vi "9. CoffeeMaker Documentation.vi"(6 "Simulation":cluster{"Water":dbl, "Coffee":dbl, "Milk":dbl} caption="Wasser" {"Milk" step=1.0 scale=0.0..100.0; "Water" step=1.0 scale=0.0..100.0; "Coffee" step=1.0 scale=0.0..100.0}, 7 "Power Switch":bool, 11 "Coffee Selection":T2 caption="Selection" {"Type" min=0 max=2 step=1 scale=0.0..2.0}) -> (0 "error out":errorcluster, 3 "Display":T1 {"Coffee" scale=0.0..80.0; "Brewing Chamber" scale=0.0..80.0})   [LabVIEW 2018]
doc: "Coffee Machine Version 1.0: final solution. Extensive documentation and VI appearance added"
uses:
  Controls/States.ctl
  <vilib>/Utility/miscctls.llb/LVMinMaxIncTypeDef.ctl
  <vilib>/Utility/file.llb/Read Delimited Spreadsheet (DBL).vi
  <vilib>/Utility/file.llb/Read Delimited Spreadsheet (string).vi
  <vilib>/Utility/file.llb/Write Delimited Spreadsheet (DBL).vi
panel:
  out "s? t:f":enum16{"next state", "current state"}(ring)
  # "CLD Coffee Machine v1.0"
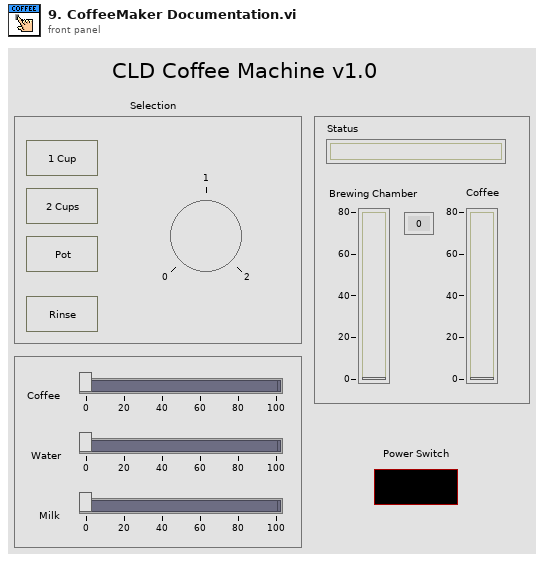
[diagram p1: front panel]
types:
  T1 = cluster{"Brewing Chamber":i8, "Coffee":i8, "Status":string, "Remaining Time:":i32}
  T2 = cluster{"1 Cup":bool, "2 Cups":bool, "Pot":bool, "Rinse":bool, "Type":i8}
  T3 = cluster{"Status":refnum<vi>, "Brewing Chamber":refnum<vi>, "Coffee":refnum<vi>, "Power Switch":refnum<vi>}
  T4 = enum8{"Enabled", "Disabled", "Disabled and Grayed Out"}
  T5 = typedef "LVMinMaxIncTypeDef.ctl" = cluster{"Minimum":dbl, "Maximum":dbl, "Increment":dbl}
  T6 = typedef "States.ctl" = enum16{"Initialize", "Set Language", "Wait for Power On", "Heat up", "Check and Wait for Water", "Rinsing", "Check Resources", "User Input", "Grinding", "Boiling", "Pouring", "Rinse before Stop", "Write Data", "Stop"}
  T7 = cluster{"Coffee":refnum<vi>, "Water":refnum<vi>, "Milk":refnum<vi>}
  T8 = cluster{"Coffee Selection":refnum<vi>, "1 Cup":refnum<vi>, "2 Cups":refnum<vi>, "Pot":refnum<vi>, "Rinse":refnum<vi>, "Type":refnum<vi>}
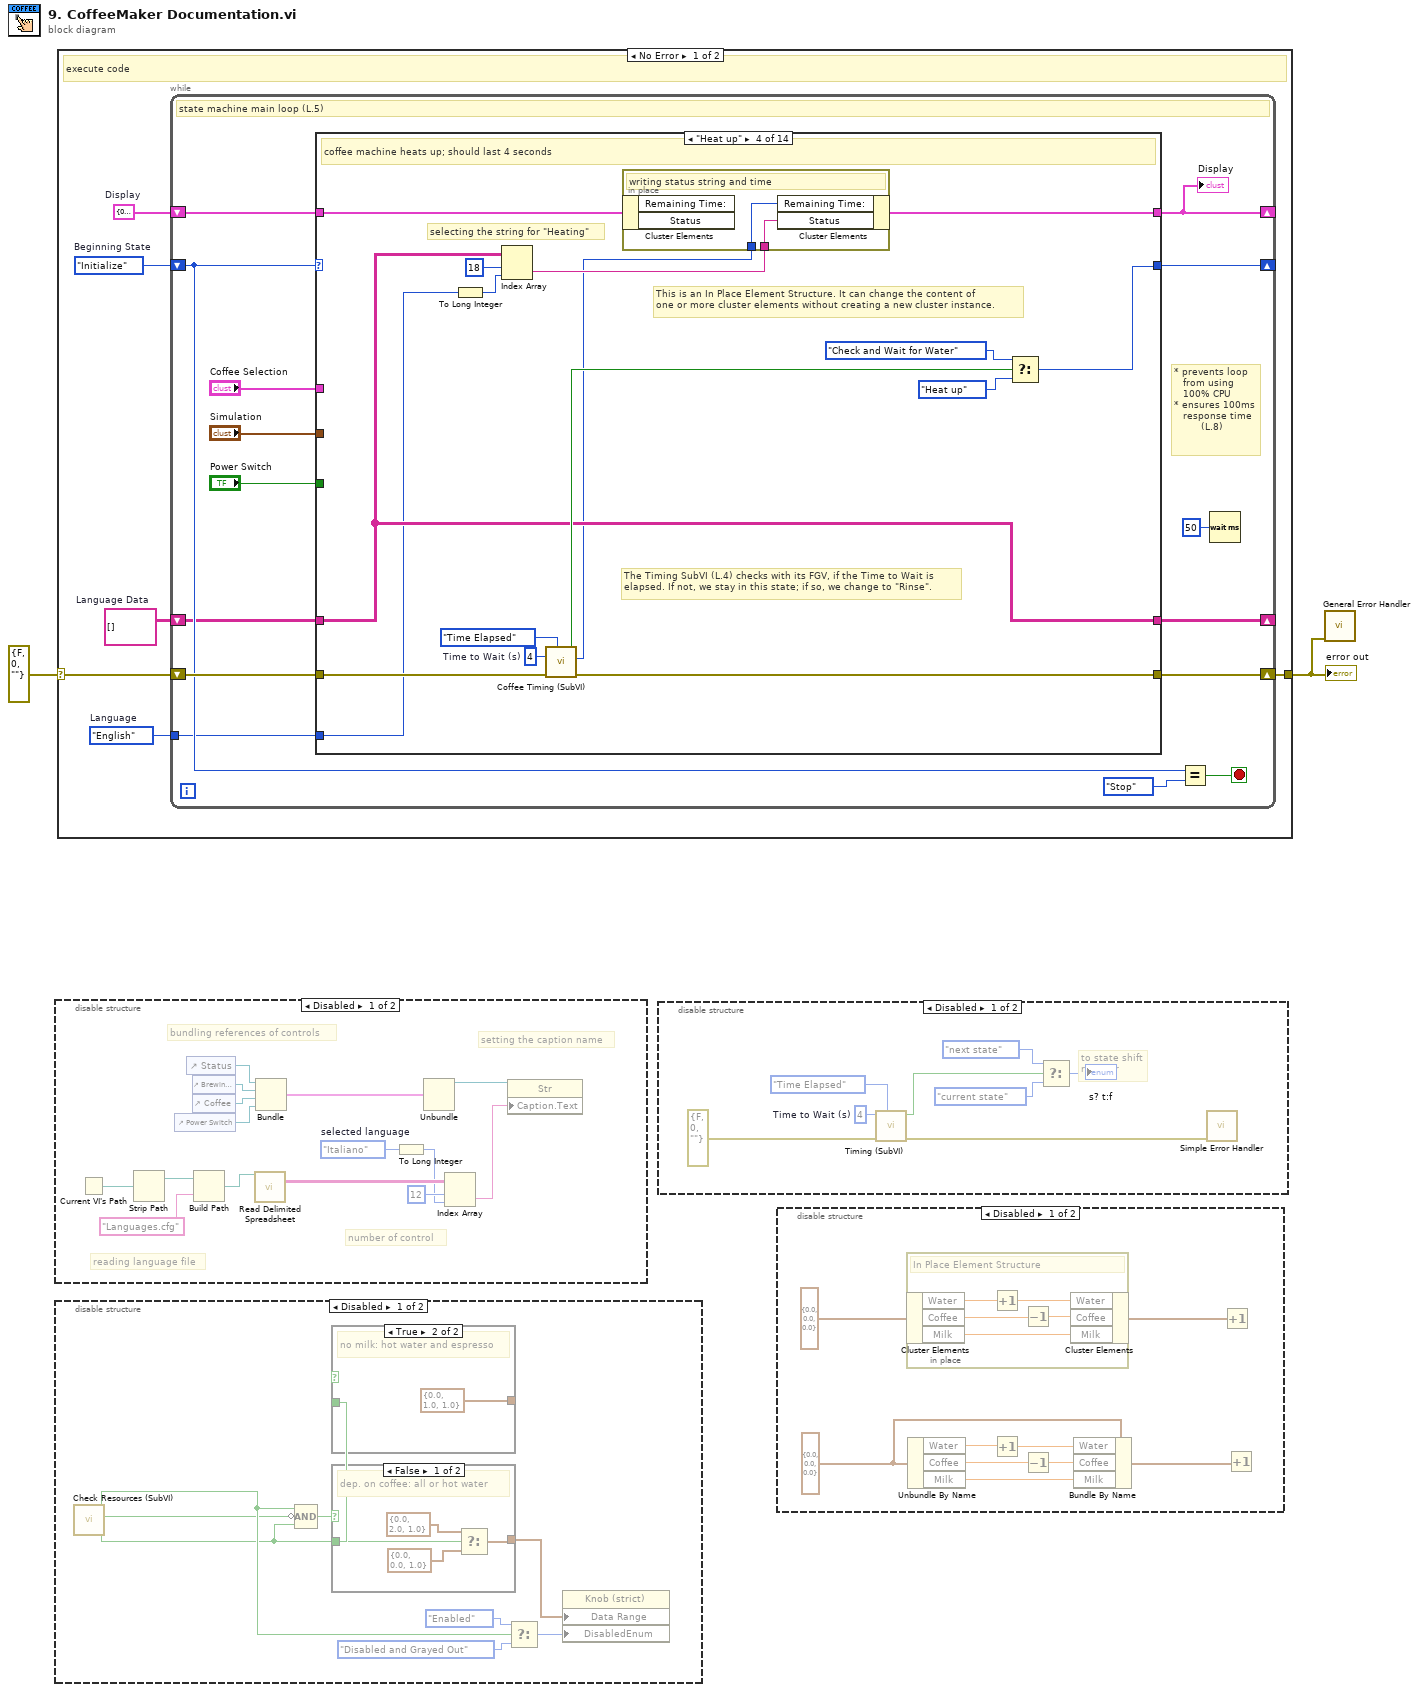
[diagram p0: block diagram]
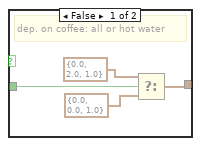
[diagram p3: hidden frame]
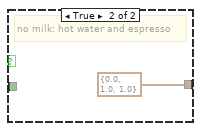
[diagram p4: hidden frame]
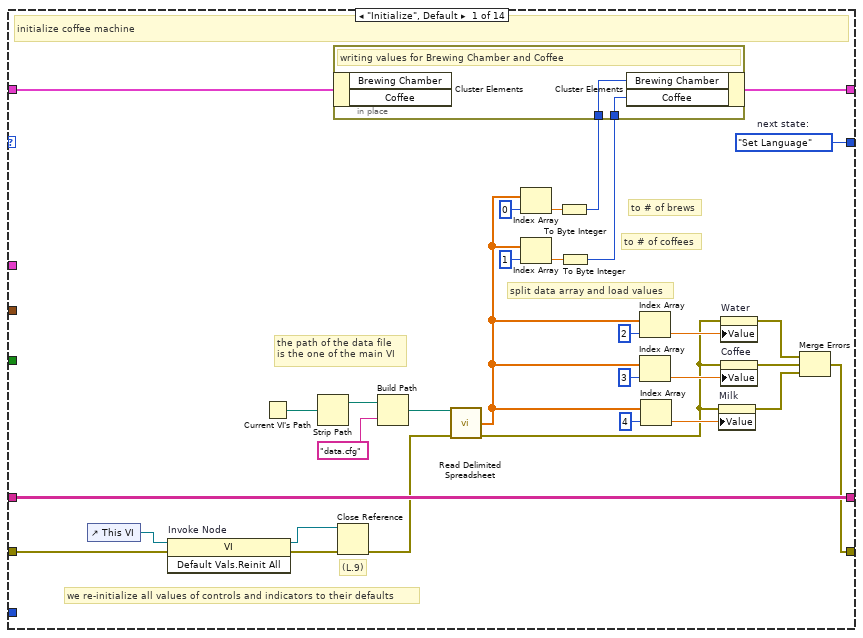
[diagram p8: hidden frame]
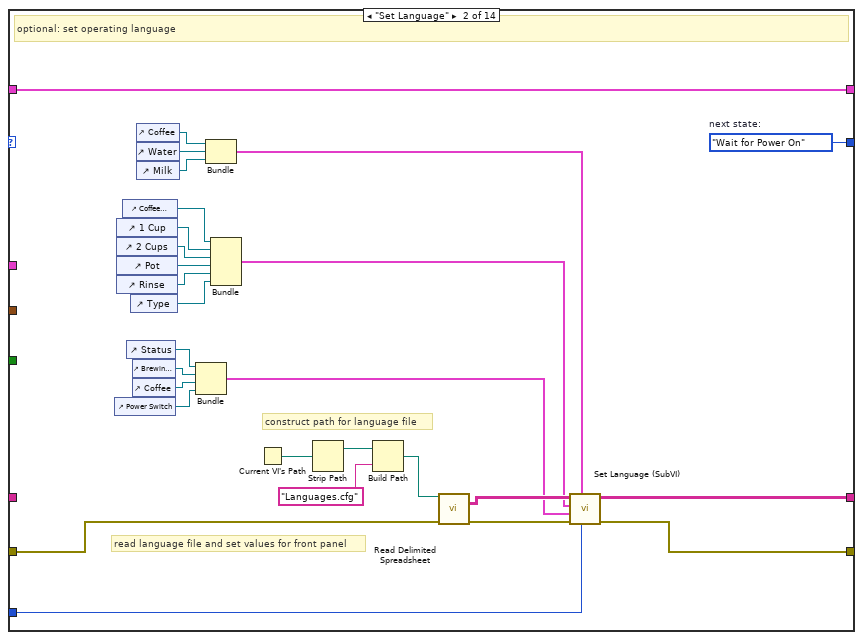
[diagram p9: hidden frame]
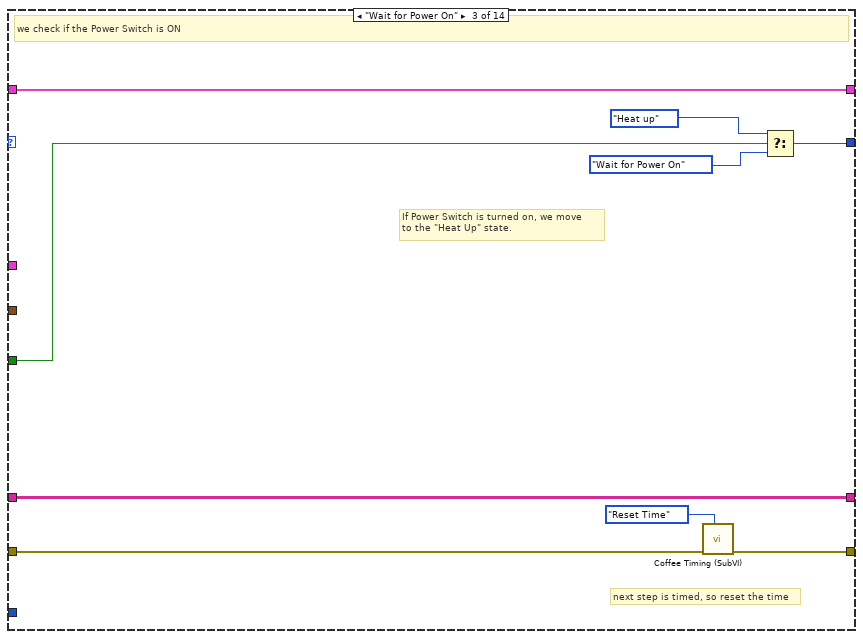
[diagram p10: hidden frame]
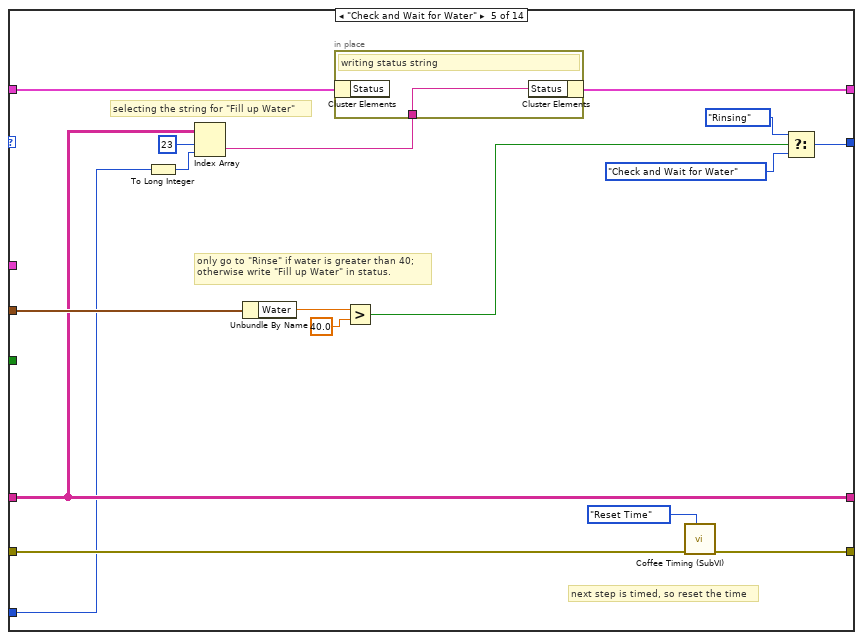
[diagram p11: hidden frame]
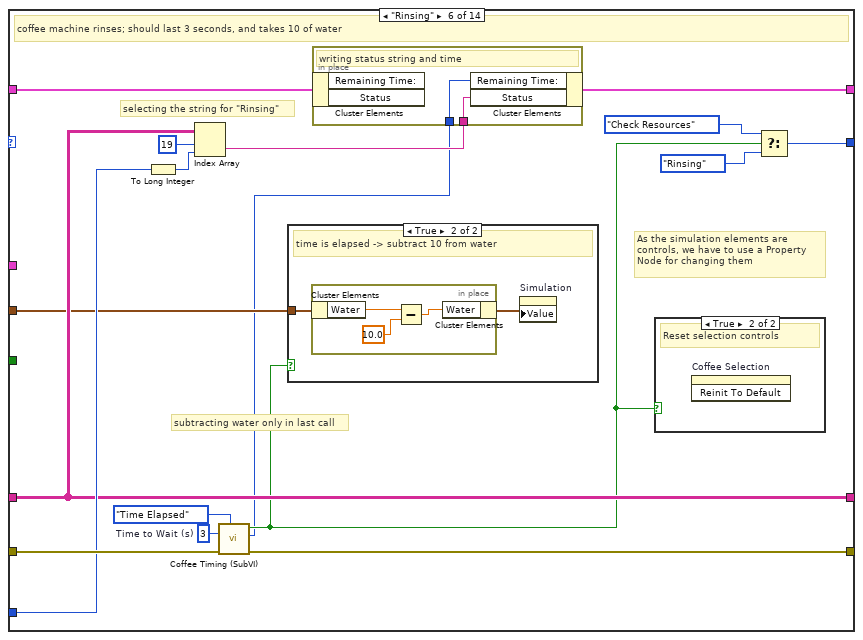
[diagram p12: hidden frame]
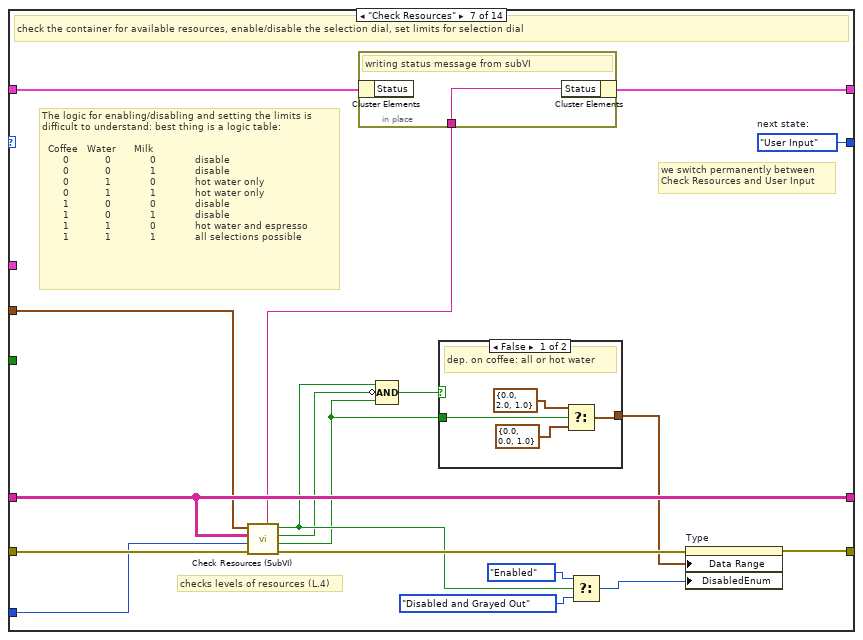
[diagram p15: hidden frame]
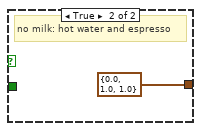
[diagram p16: hidden frame]
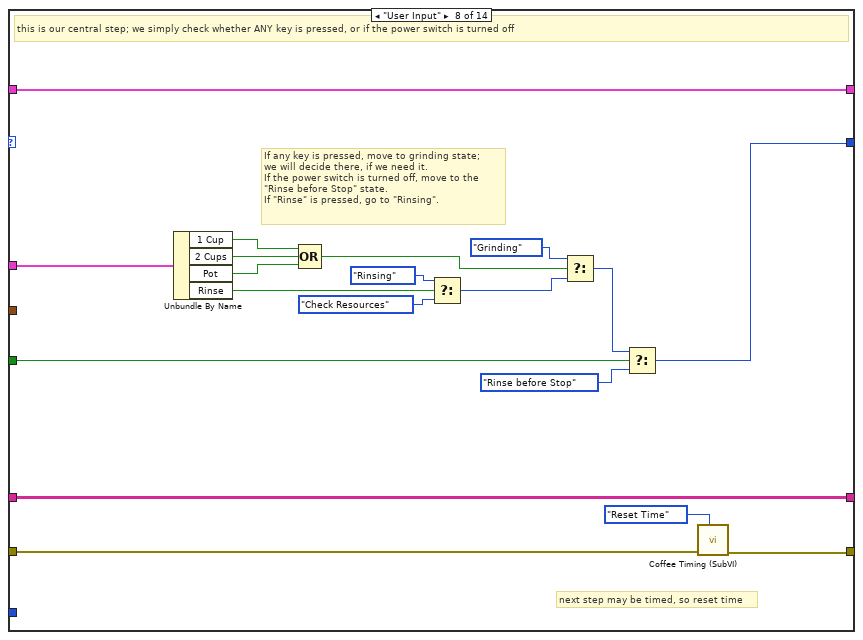
[diagram p17: hidden frame]
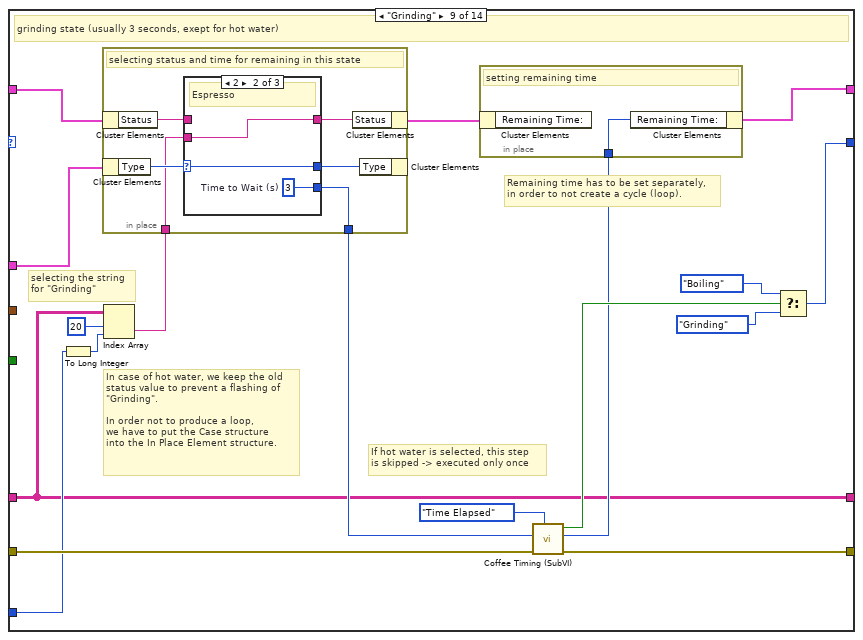
[diagram p18: hidden frame]
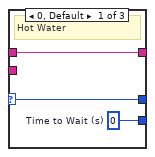
[diagram p19: hidden frame]
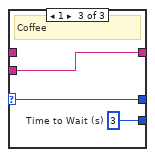
[diagram p20: hidden frame]
diagram:
  n1 = disable-structure shown="Disabled" {
    frame Disabled {
      w5 = enum16{"English", "Deutsch", "Italiano"}."Italiano"  # selected language
      # "setting the caption name"
      # "number of control"
      # "reading language file"
      # "bundling references of controls"
      n2 = Current VI's Path() -> (path=w11:path)
      n3 = Strip Path(path=w11) -> (stripped path=w10:path)  [unwired: 1 out]
      n4 = control-ref of="Power Switch"() -> (w17:refnum<vi>)
      n5 = control-ref of="Status"() -> (w14:refnum<vi>)
      n6 = control-ref of="Brewing Chamber"() -> (w15:refnum<vi>)
      n7 = control-ref of="Coffee"() -> (w16:refnum<vi>)
      n8 = Build Path(base path=w10, name or relative path="Languages.cfg") -> (appended path=w8:path)
      n9 = call-poly <vilib>:"Read Delimited Spreadsheet.vi"("file path (dialog if empty)"=w8) -> ("all rows"=w7:string[][])  [unwired: 9 in, 5 out]
      n10 = Bundle("Status"=w14, "Brewing Chamber"=w15, "Coffee"=w16, "Power Switch"=w17) -> (w13:T3)  [unwired: 1 in]
      n11 = To Long Integer(number=w5) -> (32bit integer=w4:i32)
      n12 = Unbundle(w13) -> ("Status"=w12:refnum<vi>)  [unwired: 3 out]
      n13 = Index Array(array=w7, index (row)=12, index (col)=w4) -> (element=w3:string)
      n14 = property class="Str"(reference=w12, "Caption.Text"=w3) -> ()  [unwired: 1 in, 2 out]
    }
    frame Enabled {
    }
  }
  n15 = disable-structure shown="Disabled" {
    frame Disabled {
      n16 = call "Check Resources (SubVI).vi"() -> ("Coffee ok?"=w18:bool, "Milk ok?"=w19:bool, "Water ok?"=w20:bool)  [unwired: 7 in, 2 out]
      n17 = Compound Arithmetic op=AND(w20, invert w19, w18) -> (w22:bool)
      n18 = case shown="True" {
        selector: _ -> [_ _]
        tunnel: w18 -> [w27 _]
        tunnel: [w26 T5 {"Minimum"=0.0, "Maximum"=1.0, "Increment"=1.0} ("Data Entry Limits")] -> _
        frame False {
          # "dep. on coffee: all or hot water"
          n19 = Select(t=T5 {"Minimum"=0.0, "Maximum"=2.0, "Increment"=1.0} ("Data Entry Limits"), s=w27, f=T5 {"Minimum"=0.0, "Maximum"=0.0, "Increment"=1.0} ("Data Entry Limits")) -> (s? t:f=w26:T5)
        }
        frame True {
          # "no milk: hot water and espresso"
        }
      }
      n20 = case shown="False" w22 {
        tunnel: w18 -> [w32 _]
        tunnel: [w31 T5 {"Minimum"=0.0, "Maximum"=1.0, "Increment"=1.0} ("Data Entry Limits")] -> w21
        frame False {
          # "dep. on coffee: all or hot water"
          n21 = Select(t=T5 {"Minimum"=0.0, "Maximum"=2.0, "Increment"=1.0} ("Data Entry Limits"), s=w32, f=T5 {"Minimum"=0.0, "Maximum"=0.0, "Increment"=1.0} ("Data Entry Limits")) -> (s? t:f=w31:T5)
        }
        frame True {
          # "no milk: hot water and espresso"
        }
      }
      n22 = Select(t=T4."Enabled" ("Disabled"), s=w20, f=T4."Disabled and Grayed Out" ("Disabled")) -> (s? t:f=w23:T4)
      n23 = property on="Property Node" class="Knob (strict)"("Data Range"=w21, "DisabledEnum"=w23) -> ()  [unwired: 2 in, 2 out]
    }
    frame Enabled {
    }
  }
  n24 = case shown="No Error" errorcluster {"status"=FALSE, "code"=0, "source"=""} ("error IO") {
    selector: errorcluster {"status"=FALSE, "code"=0, "source"=""} ("error IO") -> [w40 w370]
    tunnel: [w41 w370] -> w2
    frame No Error {
      w36 = T1 {"Brewing Chamber"=0, "Coffee"=0, "Status"="", "Remaining Time:"=0}  # Display
      w37 = enum16{"English", "Deutsch", "Italiano"}."English"  # Language
      w38 = string[][] []  # Language Data
      w39 = States."Initialize"  # Beginning State
      # "execute code"
      n25 = while {
        shift-right: [w53] -> _
        shift-left: w39 -> [w52]
        shift-right: [w46] -> _
        shift-left: w38 -> [w45]
        shift-right: [w42] -> _
        shift-left: w36 -> [w49]
        shift-right: [w56] -> w41
        shift-left: w40 -> [w55]
        tunnel: w37 -> [w43]
        stop <- w50 stop-if-true
        # "* prevents loop\n   from using\n   100% CPU\n* ensures 100ms\n   response time\n         (L.8)"
        # "state machine main loop (L.5)"
        n26 = case shown="\"Heat up\"" w52 {
          tunnel: [w76 w110 w121 w141 w152 w178 w194 w227 w245 w276 w289 w337 w358 w366] -> w56
          tunnel: w55 -> [w87 w111 w122 w142 w153 w179 w204 w228 w246 w277 w299 w338 w359 w366]
          tunnel: "Power Switch" -> [_ _ w126 _ _ _ _ w225 _ _ _ _ _ _]
          tunnel: [w86 w108 w125 w138 w159 w175 w198 w224 w242 w272 w296 w334 States."Stop" ("f") States."Stop" ("f")] -> w53
          tunnel: [w65 w107 w119 w133 w145 w171 w199 w215 w235 w278 w300 w331 w356 w368] -> w42
          tunnel: w49 -> [w66 w107 w119 w134 w151 w172 w201 w215 w247 w279 w301 w332 w356 w368]
          tunnel: "Coffee Selection" -> [_ _ _ _ _ _ _ w223 w239 _ w291 _ _ _]
          tunnel: "Simulation" -> [_ _ _ _ w158 w165 w202 _ _ _ w292 w326 w357 _]
          tunnel: [w85 w109 w118 w132 w148 w167 w203 w229 w231 w266 w286 w327 w364 w367] -> w46
          tunnel: w45 -> [w85 _ w118 w132 w148 w167 w203 w229 w231 w266 w286 w327 w364 w367]
          tunnel: w43 -> [_ w94 _ w129 w147 w168 w187 _ w232 w265 w285 w328 _ _]
          frame "Initialize", Default {
            w86 = States."Set Language"  # next state:
            # "to # of coffees"
            # "to # of brews"
            # "(L.9)"
            # "split data array and load values"
            # "the path of the data file \nis the one of the main VI"
            # "we re-initialize all values of controls and indicators to their defaults"
            # "initialize coffee machine"
            n27 = control-ref of="This VI"() -> (w63:refnum<vi>)
            n28 = invoke on="Invoke Node" class="VI" method="Default Vals.Reinit All"(reference=w63, error in=w87) -> (reference out=w62:refnum<vi>, error out=w61:errorcluster)  [unwired: 1 in, 1 out]
            n29 = Current VI's Path() -> (path=w83:path)
            n30 = Strip Path(path=w83) -> (stripped path=w82:path)  [unwired: 1 out]
            n31 = Close Reference(reference=w62, error in (no error)=w61) -> (error out=w84:errorcluster)
            n32 = Build Path(base path=w82, name or relative path="data.cfg") -> (appended path=w80:path)
            n33 = call-poly <vilib>:"Read Delimited Spreadsheet.vi"("file path (dialog if empty)"=w80, "error in (no error)"=w84) -> ("first row"=w79:dbl[], "error out"=w64:errorcluster)  [unwired: 8 in, 4 out]
            n34 = Index Array "Index Array"(array=w79, index=0) -> (element=w60:dbl)
            n35 = Index Array(array=w79, index=1) -> (element=w58:dbl)
            n36 = To Byte Integer(number=w60) -> (8bit integer=w59:i8)
            n37 = To Byte Integer(number=w58) -> (8bit integer=w57:i8)
            n38 = in-place {
              in-place-border: w59 -> [w89]
              in-place-border: w57 -> [w88]
              # "writing values for Brewing Chamber and Coffee"
              n39 = in-place-cluster #1(w66) -> ()  [unwired: 2 out]
              n40 = in-place-cluster #1("Brewing Chamber"=w89, "Coffee"=w88) -> (w65:T1)
            }
            n41 = Index Array(array=w79, index=2) -> (element=w70:dbl)
            n42 = Index Array(array=w79, index=3) -> (element=w68:dbl)
            n43 = Index Array(array=w79, index=4) -> (element=w78:dbl)
            n44 = property on="Milk" class="Slide (strict)"(error in=w64, "Value"=w78) -> (error out=w77:errorcluster)  [unwired: 1 in, 1 out]
            n45 = property on="Water" class="Slide (strict)"(error in=w64, "Value"=w70) -> (error out=w69:errorcluster)  [unwired: 1 in, 1 out]
            n46 = property on="Coffee" class="Slide (strict)"(error in=w64, "Value"=w68) -> (error out=w67:errorcluster)  [unwired: 1 in, 1 out]
            n47 = Merge Errors(w69, w67, w77) -> (w76:errorcluster)
          }
          frame "Set Language" {
            w108 = States."Wait for Power On"  # next state:
            # "construct path for language file"
            # "read language file and set values for front panel"
            # "optional: set operating language"
            n48 = control-ref of="Power Switch"() -> (w97:refnum<vi>)
            n49 = control-ref of="1 Cup"() -> (w105:refnum<vi>)
            n50 = control-ref of="2 Cups"() -> (w104:refnum<vi>)
            n51 = control-ref of="Pot"() -> (w103:refnum<vi>)
            n52 = control-ref of="Rinse"() -> (w102:refnum<vi>)
            n53 = control-ref of="Coffee Selection"() -> (w106:refnum<vi>)
            n54 = control-ref of="Status"() -> (w100:refnum<vi>)
            n55 = control-ref of="Type"() -> (w101:refnum<vi>)
            n56 = control-ref of="Brewing Chamber"() -> (w99:refnum<vi>)
            n57 = control-ref of="Coffee"() -> (w98:refnum<vi>)
            n58 = control-ref of="Coffee"() -> (w93:refnum<vi>)
            n59 = control-ref of="Water"() -> (w92:refnum<vi>)
            n60 = control-ref of="Milk"() -> (w91:refnum<vi>)
            n61 = Bundle("Status"=w100, "Brewing Chamber"=w99, "Coffee"=w98, "Power Switch"=w97) -> (w95:T3)  [unwired: 1 in]
            n62 = Bundle("Coffee"=w93, "Water"=w92, "Milk"=w91) -> (w90:T7)  [unwired: 1 in]
            n63 = Bundle("Coffee Selection"=w106, "1 Cup"=w105, "2 Cups"=w104, "Pot"=w103, "Rinse"=w102, "Type"=w101) -> (w96:T8)  [unwired: 1 in]
            n64 = Current VI's Path() -> (path=w112:path)
            n65 = Strip Path(path=w112) -> (stripped path=w113:path)  [unwired: 1 out]
            n66 = Build Path(base path=w113, name or relative path="Languages.cfg") -> (appended path=w115:path)
            n67 = call-poly <vilib>:"Read Delimited Spreadsheet.vi"("file path (dialog if empty)"=w115, "error in (no error)"=w111) -> ("all rows"=w117:string[][], "error out"=w116:errorcluster)  [unwired: 8 in, 4 out]
            n68 = call "Set Language (SubVI).vi"("Language (English)"=w94, "Simulation \nReferences"=w90, "error in (no error)"=w116, "Status\nReferences"=w95, "Selection \nReferences"=w96, "Language Data"=w117) -> ("error out"=w110:errorcluster, "Language Data Out"=w109:string[][])  [unwired: 4 in]
          }
          frame "Wait for Power On" {
            # "next step is timed, so reset the time"
            # "If Power Switch is turned on, we move\nto the \"Heat Up\" state."
            # "we check if the Power Switch is ON"
            n69 = call "Coffee Timing (SubVI).vi"("Function"=enum16{"Reset Time", "Time Elapsed"}."Reset Time", "error in (no error)"=w122) -> ("error out"=w121:errorcluster)  [unwired: 7 in, 2 out]
            n70 = Select(t=States."Heat up" ("Beginning State"), s=w126, f=States."Wait for Power On") -> (s? t:f=w125:T6)
          }
          frame "Heat up" {
            w139 = 4  # Time to Wait (s)
            # "selecting the string for \"Heating\""
            # "This is an In Place Element Structure. It can change the content of\none or more cluster elements without creating a new cluster instance."
            # "The Timing SubVI (L.4) checks with its FGV, if the Time to Wait is\nelapsed. If not, we stay in this state; if so, we change to \"Rinse\"."
            # "coffee machine heats up; should last 4 seconds"
            n71 = To Long Integer(number=w129) -> (32bit integer=w130:i32)
            n72 = Index Array "Index Array"(array=w132, index (row)=18, index (col)=w130) -> (element=w128:string)
            n73 = call "Coffee Timing (SubVI).vi"("Function"=enum16{"Reset Time", "Time Elapsed"}."Time Elapsed", "error in (no error)"=w142, "Time to Wait (s)"=w139) -> ("error out"=w141:errorcluster, "Remaining Time"=w127:i32, "Time elapsed ?"=w135:bool)  [unwired: 6 in]
            n74 = in-place {
              in-place-border: w128 -> [w144]
              in-place-border: w127 -> [w143]
              # "writing status string and time"
              n75 = in-place-cluster #2(w134) -> ()  [unwired: 2 out]
              n76 = in-place-cluster #2("Remaining Time:"=w143, "Status"=w144) -> (w133:T1)
            }
            n77 = Select(t=States."Check and Wait for Water" ("Beginning State"), s=w135, f=States."Heat up" ("Beginning State")) -> (s? t:f=w138:T6)
          }
          frame "Check and Wait for Water" {
            # "next step is timed, so reset the time"
            # "only go to \"Rinse\" if water is greater than 40;\notherwise write \"Fill up Water\" in status."
            # "selecting the string for \"Fill up Water\""
            n78 = To Long Integer(number=w147) -> (32bit integer=w149:i32)
            n79 = Index Array "Index Array"(array=w148, index (row)=23, index (col)=w149) -> (element=w146:string)
            n80 = Unbundle By Name(w158) -> ("Water"=w157:dbl)
            n81 = in-place {
              in-place-border: w146 -> [w162]
              # "writing status string"
              n82 = in-place-cluster #3(w151) -> ()  [unwired: 1 out]
              n83 = in-place-cluster #3("Status"=w162) -> (w145:T1)
            }
            n84 = Greater?(x=w157, y=40.0) -> (0:w155:bool)
            n85 = call "Coffee Timing (SubVI).vi"("Function"=enum16{"Reset Time", "Time Elapsed"}."Reset Time", "error in (no error)"=w153) -> ("error out"=w152:errorcluster)  [unwired: 7 in, 2 out]
            n86 = Select(t=States."Rinsing" ("f"), s=w155, f=States."Check and Wait for Water") -> (s? t:f=w159:T6)
          }
          frame "Rinsing" {
            w176 = 3  # Time to Wait (s)
            # "subtracting water only in last call"
            # "As the simulation elements are\ncontrols, we have to use a Property \nNode for changing them"
            # "selecting the string for \"Rinsing\""
            # "coffee machine rinses; should last 3 seconds, and takes 10 of water"
            n87 = To Long Integer(number=w168) -> (32bit integer=w169:i32)
            n88 = Index Array "Index Array"(array=w167, index (row)=19, index (col)=w169) -> (element=w166:string)
            n89 = call "Coffee Timing (SubVI).vi"("Function"=enum16{"Reset Time", "Time Elapsed"}."Time Elapsed", "error in (no error)"=w179, "Time to Wait (s)"=w176) -> ("error out"=w178:errorcluster, "Remaining Time"=w163:i32, "Time elapsed ?"=w164:bool)  [unwired: 6 in]
            n90 = case shown="True" w164 {
              tunnel: w165 -> [_ w181]
              frame False {
                # "time is running ..."
              }
              frame True {
                # "time is elapsed -> subtract 10 from water"
                n91 = in-place {
                  n92 = in-place-cluster #4(w181) -> ("Water"=w184:dbl)
                  n93 = Subtract(x=w184, y=10.0) -> (x-y=w182:dbl)
                  n94 = in-place-cluster #4("Water"=w182) -> (w180:cluster{"Water":dbl, "Coffee":dbl, "Milk":dbl})
                }
                n95 = property on="Simulation" class="Clust (strict)"("Value"=w180) -> ()  [unwired: 2 in, 2 out]
              }
            }
            n96 = in-place {
              in-place-border: w166 -> [w186]
              in-place-border: w163 -> [w185]
              # "writing status string and time"
              n97 = in-place-cluster #5(w172) -> ()  [unwired: 2 out]
              n98 = in-place-cluster #5("Remaining Time:"=w185, "Status"=w186) -> (w171:T1)
            }
            n99 = case shown="True" w164 {
              frame False {
              }
              frame True {
                # "Reset selection controls"
                n100 = invoke on="Coffee Selection" class="Clust (strict)" method="Reinit To Default"() -> ()  [unwired: 3 in, 3 out]
              }
            }
            n101 = Select(t=States."Check Resources" ("Beginning State"), s=w164, f=States."Rinsing" ("Beginning State")) -> (s? t:f=w175:T6)
          }
          frame "Check Resources" {
            w198 = States."User Input"  # next state:
            # "checks levels of resources (L.4)"
            # "The logic for enabling/disabling and setting the limits is \ndifficult to understand: best thing is a logic table:\n\n  Coffee   Water      Milk\n       0            0             0             disable\n       0            0             1             disable\n       0            1             0             hot water only\n       0            1             1             hot water only\n       1            0             0             disable\n       1            0             1             disable\n       1            1             0             hot water and espresso\n       1            1             1             all selections possible"
            # "we switch permanently between \nCheck Resources and User Input"
            # "check the container for available resources, enable/disable the selection dial, set limits for selection dial"
            n102 = call "Check Resources (SubVI).vi"("error in (no error)"=w204, "Language"=w187, "Language Data"=w203, "Simulation"=w202) -> ("error out"=w195:errorcluster, "Coffee ok?"=w189:bool, "Milk ok?"=w191:bool, "Water ok?"=w192:bool, "Status Message"=w200:string)  [unwired: 3 in]
            n103 = in-place {
              in-place-border: w200 -> [w210]
              # "writing status message from subVI"
              n104 = in-place-cluster #6(w201) -> ()  [unwired: 1 out]
              n105 = in-place-cluster #6("Status"=w210) -> (w199:T1)
            }
            n106 = Compound Arithmetic op=AND(w192, invert w191, w189) -> (w190:bool)
            n107 = case shown="False" w190 {
              tunnel: w189 -> [w206 _]
              tunnel: [w205 T5 {"Minimum"=0.0, "Maximum"=1.0, "Increment"=1.0} ("Data Entry Limits")] -> w188
              frame False {
                # "dep. on coffee: all or hot water"
                n108 = Select(t=T5 {"Minimum"=0.0, "Maximum"=2.0, "Increment"=1.0} ("Data Entry Limits"), s=w206, f=T5 {"Minimum"=0.0, "Maximum"=0.0, "Increment"=1.0} ("Data Entry Limits")) -> (s? t:f=w205:T5)
              }
              frame True {
                # "no milk: hot water and espresso"
              }
            }
            n109 = Select(t=T4."Enabled" ("Disabled"), s=w192, f=T4."Disabled and Grayed Out" ("Disabled")) -> (s? t:f=w193:T4)
            n110 = property on="Type" class="Knob (strict)"(error in=w195, "Data Range"=w188, "DisabledEnum"=w193) -> (error out=w194:errorcluster)  [unwired: 1 in, 1 out]
          }
          frame "User Input" {
            # "If any key is pressed, move to grinding state; \nwe will decide there, if we need it.\nIf the power switch is turned off, move to the \n\"Rinse before Stop\" state.\nIf \"Rinse\" is pressed, go to \"Rinsing\"."
            # "next step may be timed, so reset time"
            # "this is our central step; we simply check whether ANY key is pressed, or if the power switch is turned off"
            n111 = Unbundle By Name(w223) -> ("1 Cup"=w222:bool, "2 Cups"=w221:bool, "Pot"=w220:bool, "Rinse"=w214:bool)
            n112 = Compound Arithmetic op=OR(w222, w221, w220) -> (w217:bool)
            n113 = Select(t=States."Rinsing", s=w214, f=States."Check Resources" ("t")) -> (s? t:f=w211:T6)
            n114 = Select(t=States."Grinding", s=w217, f=w211) -> (s? t:f=w218:T6)
            n115 = Select(t=w218, s=w225, f=States."Rinse before Stop") -> (s? t:f=w224:T6)
            n116 = call "Coffee Timing (SubVI).vi"("Function"=enum16{"Reset Time", "Time Elapsed"}."Reset Time", "error in (no error)"=w228) -> ("error out"=w227:errorcluster)  [unwired: 7 in, 2 out]
          }
          frame "Grinding" {
            # "selecting the string \nfor \"Grinding\""
            # "Remaining time has to be set separately,\nin order to not create a cycle (loop)."
            # "In case of hot water, we keep the old\nstatus value to prevent a flashing of\n\"Grinding\".\n\nIn order not to produce a loop,\nwe have to put the Case structure\ninto the In Place Element structure."
            # "If hot water is selected, this step\nis skipped -> executed only once"
            # "grinding state (usually 3 seconds, exept for hot water)"
            n117 = To Long Integer(number=w232) -> (32bit integer=w233:i32)
            n118 = Index Array "Index Array"(array=w231, index (row)=20, index (col)=w233) -> (element=w230:string)
            n119 = in-place {
              in-place-border: [w251] -> w238
              in-place-border: w230 -> [w249]
              # "selecting status and time for remaining in this state"
              n120 = in-place-cluster #7(w247) -> ("Status"=w253:string)
              n121 = in-place-cluster #8(w239) -> ("Type"=w254:i8)
              n122 = case shown="2" w254 {
                selector: w254 -> [w255 w259 w262]
                tunnel: [w257 w260 w263] -> w251
                tunnel: [w256 w258 w261] -> w252
                tunnel: w253 -> [w256 _ _]
                tunnel: [w255 w259 w262] -> w250
                tunnel: w249 -> [_ w258 w261]
                frame 0, Default {
                  w257 = 0  # Time to Wait (s)
                  # "Hot Water"
                }
                frame 2 {
                  w260 = 3  # Time to Wait (s)
                  # "Espresso"
                }
                frame 1 {
                  w263 = 3  # Time to Wait (s)
                  # "Coffee"
                }
              }
              n123 = in-place-cluster #7("Status"=w252) -> (w237:T1)
              n124 = in-place-cluster #8("Type"=w250) -> ()  [unwired: 1 out]
            }
            n125 = call "Coffee Timing (SubVI).vi"("Function"=enum16{"Reset Time", "Time Elapsed"}."Time Elapsed", "error in (no error)"=w246, "Time to Wait (s)"=w238) -> ("error out"=w245:errorcluster, "Remaining Time"=w236:i32, "Time elapsed ?"=w243:bool)  [unwired: 6 in]
            n126 = in-place {
              in-place-border: w236 -> [w248]
              # "setting remaining time"
              n127 = in-place-cluster #9(w237) -> ()  [unwired: 1 out]
              n128 = in-place-cluster #9("Remaining Time:"=w248) -> (w235:T1)
            }
            n129 = Select(t=States."Boiling" ("Beginning State"), s=w243, f=States."Grinding") -> (s? t:f=w242:T6)
          }
          frame "Boiling" {
            w275 = 3  # Time to Wait (s)
            # "selecting the string for \"Boiling\""
            # "nothing special happens here"
            # "boiling state (3 seconds)"
            n130 = To Long Integer(number=w265) -> (32bit integer=w267:i32)
            n131 = Index Array "Index Array"(array=w266, index (row)=21, index (col)=w267) -> (element=w264:string)
            n132 = call "Coffee Timing (SubVI).vi"("Function"=enum16{"Reset Time", "Time Elapsed"}."Time Elapsed", "error in (no error)"=w277, "Time to Wait (s)"=w275) -> ("error out"=w276:errorcluster, "Remaining Time"=w269:i32, "Time elapsed ?"=w273:bool)  [unwired: 6 in]
            n133 = in-place {
              in-place-border: w269 -> [w281]
              in-place-border: w264 -> [w280]
              n134 = in-place-cluster #10(w279) -> ()  [unwired: 2 out]
              n135 = in-place-cluster #10("Status"=w280, "Remaining Time:"=w281) -> (w278:T1)
            }
            n136 = Select(t=States."Pouring" ("Beginning State"), s=w273, f=States."Boiling") -> (s? t:f=w272:T6)
          }
          frame "Pouring" {
            w298 = 5  # Time to Wait (s)
            # "selecting the string \nfor \"Pouring\""
            # "pouring state (5 seconds). in the final run, container values are reduced and switches are reset"
            n137 = To Long Integer(number=w285) -> (32bit integer=w287:i32)
            n138 = Index Array "Index Array"(array=w286, index (row)=22, index (col)=w287) -> (element=w284:string)
            n139 = call "Coffee Timing (SubVI).vi"("Function"=enum16{"Reset Time", "Time Elapsed"}."Time Elapsed", "error in (no error)"=w299, "Time to Wait (s)"=w298) -> ("error out"=w290:errorcluster, "Remaining Time"=w282:i32, "Time elapsed ?"=w293:bool)  [unwired: 6 in]
            n140 = case shown="True" w293 {
              tunnel: w292 -> [_ w310]
              tunnel: w291 -> [_ w311]
              tunnel: w290 -> [w303 w309]
              tunnel: [w303 w308] -> w289
              tunnel: [cluster{"coffee":i8, "chamber":i8} {"coffee"=0, "chamber"=0} ("Coffe and Chamber increase") w307] -> w283
              frame False {
                # "... time is still running ..."
              }
              frame True {
                # "writing new container values"
                # "calculates new resource container levels (L.4)"
                # "As buttons have mech \naction  \"Switch when \npressed\", they  have to \nbe released when order \nhas been processed."
                # "time is elapsed; update container values and reset switches"
                n141 = call "Subtract Resources (SubVI).vi"("error in (no error)"=w309, "Simulation in"=w310, "Coffee Selection"=w311) -> ("error out"=w305:errorcluster, "Simulation out"=w306:cluster{"Water":dbl, "Coffee":dbl, "Milk":dbl}, "Coffe and Chamber increase"=w307:cluster{"coffee":i8, "chamber":i8})  [unwired: 6 in]
                n142 = property on="Simulation" class="Clust (strict)"(error in=w305, "Value"=w306) -> (error out=w304:errorcluster)  [unwired: 1 in, 1 out]
                n143 = invoke on="Coffee Selection" class="Clust (strict)" method="Reinit To Default"(error in=w304) -> (error out=w308:errorcluster)  [unwired: 2 in, 2 out]
              }
            }
            n144 = in-place {
              in-place-border: w282 -> [w320]
              in-place-border: w283 -> [w319]
              in-place-border: w284 -> [w312]
              n145 = in-place-cluster #11(w301) -> ("Brewing Chamber"=w318:i8, "Coffee"=w316:i8)  [unwired: 2 out]
              n146 = Unbundle By Name(w319) -> ("chamber"=w313:i8, "coffee"=w314:i8)
              n147 = Add(x=w318, y=w313) -> (x+y=w317:i8)
              n148 = Add(x=w316, y=w314) -> (x+y=w315:i8)
              n149 = in-place-cluster #11("Status"=w312, "Remaining Time:"=w320, "Brewing Chamber"=w317, "Coffee"=w315) -> (w300:T1)
            }
            n150 = Select(t=States."Check Resources" ("Beginning State"), s=w293, f=States."Pouring") -> (s? t:f=w296:T6)
          }
          frame "Rinse before Stop" {
            w335 = 3  # Time to Wait (s)
            # "subtracting water only in last call"
            # "selecting the string for \"Rinsing\""
            # "coffee machine rinses before stopping; should last 3 seconds, and takes 10 of water"
            n151 = To Long Integer(number=w328) -> (32bit integer=w329:i32)
            n152 = Index Array "Index Array"(array=w327, index (row)=19, index (col)=w329) -> (element=w322:string)
            n153 = call "Coffee Timing (SubVI).vi"("Function"=enum16{"Reset Time", "Time Elapsed"}."Time Elapsed", "error in (no error)"=w338, "Time to Wait (s)"=w335) -> ("error out"=w337:errorcluster, "Remaining Time"=w321:i32, "Time elapsed ?"=w324:bool)  [unwired: 6 in]
            n154 = case shown="True" w324 {
              tunnel: [w339 ""] -> w323
              tunnel: w322 -> [w339 _]
              frame False {
                # "write status"
              }
              frame True {
                # "clear status"
              }
            }
            n155 = in-place {
              in-place-border: w323 -> [w347]
              in-place-border: w321 -> [w346]
              # "writing status string"
              n156 = in-place-cluster #12(w332) -> ()  [unwired: 2 out]
              n157 = in-place-cluster #12("Status"=w347, "Remaining Time:"=w346) -> (w331:T1)
            }
            n158 = case shown="True" w324 {
              tunnel: w326 -> [_ w342]
              frame False {
                # "time is running ..."
              }
              frame True {
                # "time is elapsed -> subtract 10 from water"
                n159 = in-place {
                  n160 = in-place-cluster #13(w342) -> ("Water"=w345:dbl)
                  n161 = Subtract(x=w345, y=10.0) -> (x-y=w343:dbl)
                  n162 = in-place-cluster #13("Water"=w343) -> (w341:cluster{"Water":dbl, "Coffee":dbl, "Milk":dbl})
                }
                n163 = property on="Simulation" class="Clust (strict)"("Value"=w341) -> ()  [unwired: 2 in, 2 out]
              }
            }
            n164 = Select(t=States."Write Data" ("Beginning State"), s=w324, f=States."Rinse before Stop") -> (s? t:f=w334:T6)
          }
          frame "Write Data" {
            # "the path of the data file \nis the one of the main VI"
            # "writing the data from the status indicators"
            n165 = Unbundle By Name(w356) -> ("Brewing Chamber"=w351:i8, "Coffee"=w348:i8)
            n166 = Unbundle By Name(w357) -> ("Water"=w355:dbl, "Coffee"=w354:dbl, "Milk"=w353:dbl)
            n167 = To Double Precision Float(number=w351) -> (double precision float=w350:dbl)
            n168 = To Double Precision Float(number=w348) -> (double precision float=w349:dbl)
            n169 = Build Array(w350, w349, w355, w354, w353) -> (w352:dbl[])
            n170 = Current VI's Path() -> (path=w363:path)
            n171 = Strip Path(path=w363) -> (stripped path=w362:path)  [unwired: 1 out]
            n172 = Build Path(base path=w362, name or relative path="data.cfg") -> (appended path=w360:path)
            n173 = call-poly <vilib>:"Write Delimited Spreadsheet.vi"("file path (dialog if empty)"=w360, "1D data"=w352, "error in (no error)"=w359) -> ("error out"=w358:errorcluster)  [unwired: 11 in, 1 out]
          }
          frame "Stop" {
            # "this one is just to make sure the program stops"
          }
        }
        "Display" <- w42
        n174 = Equal?(x=w52, y=States."Stop") -> (x = y?=w50:bool)
        n175 = Wait (ms)(milliseconds to wait=u32 50) -> ()  [unwired: 1 out]
      }
    }
    frame Error {
      # "do nothing"
    }
  }
  "error out" <- w2
  n176 = disable-structure shown="Disabled" {
    frame Disabled {
      w377 = 4  # Time to Wait (s)
      # "to state shift\nregister"
      n177 = call "Timing (SubVI).vi"("Function"=enum16{"Reset Time", "Time Elapsed"}."Time Elapsed", "error in (no error)"=errorcluster {"status"=FALSE, "code"=0, "source"=""}, "Time to Wait (s)"=w377) -> ("error out"=w375:errorcluster, "Time elapsed ?"=w374:bool)  [unwired: 6 in, 1 out]
      n178 = Select(t=enum16{"next state", "current state"}."next state", s=w374, f=enum16{"next state", "current state"}."current state") -> (s? t:f=→"s? t:f":enum16{"next state", "current state"})
      n179 = call <vilib>:"Simple Error Handler.vi"("error in (no error)"=w375) -> ()  [unwired: 4 in, 5 out]
    }
    frame Enabled {
    }
  }
  n180 = disable-structure shown="Disabled" {
    frame Disabled {
      w385 = cluster{"Water":dbl, "Coffee":dbl, "Milk":dbl} {"Water"=0.0, "Coffee"=0.0, "Milk"=0.0} ("Simulation")
      n181 = in-place {
        # "In Place Element Structure"
        n182 = in-place-cluster #14(cluster{"Water":dbl, "Coffee":dbl, "Milk":dbl} {"Water"=0.0, "Coffee"=0.0, "Milk"=0.0} ("Simulation")) -> ("Water"=w392:dbl, "Coffee"=w390:dbl, "Milk"=w388:dbl)
        n183 = Increment(x=w392) -> (x+1=w391:dbl)
        n184 = Decrement(x=w390) -> (x-1=w389:dbl)
        n185 = in-place-cluster #14("Water"=w391, "Coffee"=w389, "Milk"=w388) -> (w386:cluster{"Water":dbl, "Coffee":dbl, "Milk":dbl})
      }
      n186 = Unbundle By Name(w385) -> ("Water"=w384:dbl, "Coffee"=w381:dbl, "Milk"=w380:dbl)
      n187 = Increment(x=w384) -> (x+1=w383:dbl)
      n188 = Decrement(x=w381) -> (x-1=w382:dbl)
      n189 = Bundle By Name(cluster=w385, "Water"=w383, "Coffee"=w382, "Milk"=w380) -> (w379:cluster{"Water":dbl, "Coffee":dbl, "Milk":dbl})
      n190 = Increment(x=w386) -> ()  [unwired: 1 out]
      n191 = Increment(x=w379) -> ()  [unwired: 1 out]
    }
    frame Enabled {
    }
  }
  n192 = call <vilib>:"General Error Handler.vi"("error in (no error)"=w2) -> ()  [unwired: 10 in, 5 out]
